vi "Query Capabilities (Voltage).vi"(0 "VISA resource name":refnum<visa-resource-name>, 5 "Absolute Maximums (T)":bool=TRUE, 11 "error in (no error)":errorcluster) -> (4 "VISA resource name out":refnum<visa-resource-name>, 6 "Voltage Capabilities":T1, 15 "error out":errorcluster)   [LabVIEW 2012, in "NH Research Regenerative Test Series.lvlib"]
doc: "Returns various Voltage capabilities of the module."
uses:
  <instrlib>/NH Research Regenerative Test Series/NH Research Regenerative Test Series.lvlib
  <instrlib>/NH Research Regenerative Test Series/Public/Utility/Voltage Capabilities.ctl
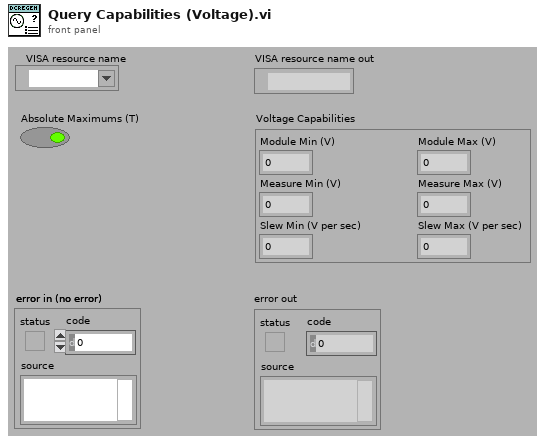
[diagram p1: front panel]
types:
  T1 = typedef "NH Research Regenerative Test Series.lvlib/Voltage Capabilities.ctl" = cluster{"Module Min (V)":dbl, "Module Max (V)":dbl, "Measure Min (V)":dbl, "Measure Max (V)":dbl, "Slew Min (V per sec)":dbl, "Slew Max (V per sec)":dbl}
  T2 = cluster{"[0]":dbl, "[1]":dbl, "[2]":dbl, "[3]":dbl, "[4]":dbl, "[5]":dbl}
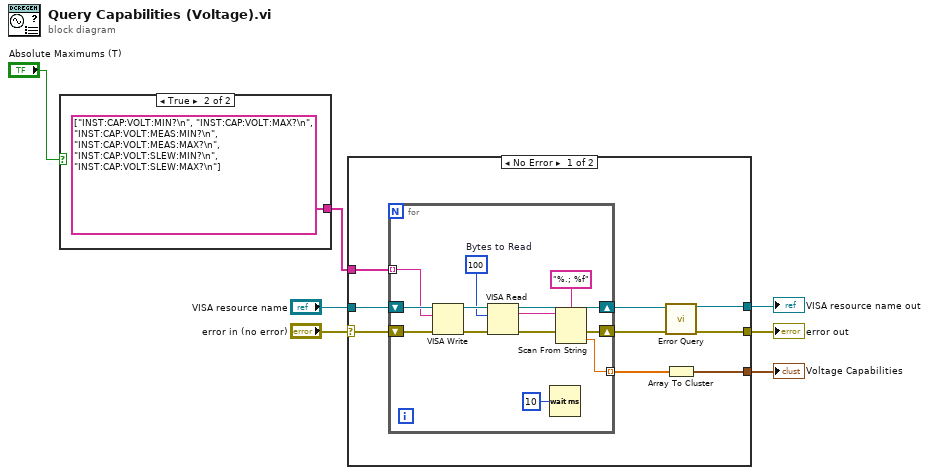
[diagram p0: block diagram]
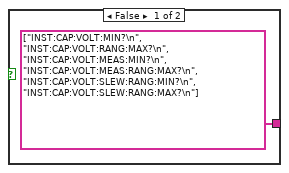
[diagram p2: hidden frame]
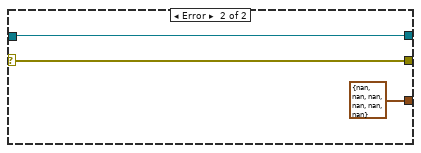
[diagram p3: hidden frame]
diagram:
  n1 = case shown="True" "Absolute Maximums (T)" {
    tunnel: [string[] ["INST:CAP:VOLT:MIN?\n", "INST:CAP:VOLT:RANG:MAX?\n", "INST:CAP:VOLT:MEAS:MIN?\n", "INST:CAP:VOLT:MEAS:RANG:MAX?\n", "INST:CAP:VOLT:SLEW:RANG:MIN?\n", "INST:CAP:VOLT:SLEW:RANG:MAX?\n"] string[] ["INST:CAP:VOLT:MIN?\n", "INST:CAP:VOLT:MAX?\n", "INST:CAP:VOLT:MEAS:MIN?\n", "INST:CAP:VOLT:MEAS:MAX?\n", "INST:CAP:VOLT:SLEW:MIN?\n", "INST:CAP:VOLT:SLEW:MAX?\n"]] -> w3
    frame False {
    }
    frame True {
    }
  }
  n2 = case shown="No Error" "error in (no error)" {
    selector: "error in (no error)" -> [w17 w34]
    tunnel: [w12 w34] -> w6
    tunnel: [w18 w33] -> w4
    tunnel: "VISA resource name" -> [w16 w33]
    tunnel: w3 -> [w15 _]
    tunnel: [w11 T1 {"Module Min (V)"=nan, "Module Max (V)"=nan, "Measure Min (V)"=nan, "Measure Max (V)"=nan, "Slew Min (V per sec)"=nan, "Slew Max (V per sec)"=nan}] -> w2
    frame No Error {
      n3 = for {
        tunnel: w15 -> [w26] mode=indexing
        tunnel: [w22] -> w14 mode=indexing
        shift-right: [w21] -> w13
        shift-left: w17 -> [w28]
        shift-right: [w20] -> w10
        shift-left: w16 -> [w27]
        w29 = u32 100  # Bytes to Read
        n4 = VISA Write(VISA resource name=w27, write buffer=w26, error in (no error)=w28) -> (VISA resource name out=w30:refnum<visa-resource-name>, error out=w31:errorcluster)  [unwired: 1 out]
        n5 = VISA Read(VISA resource name=w30, byte count=w29, error in (no error)=w31) -> (VISA resource name out=w20:refnum<visa-resource-name>, read buffer=w23:string, error out=w24:errorcluster)  [unwired: 1 out]
        n6 = Wait (ms)(milliseconds to wait=u32 10) -> ()  [unwired: 1 out]
        n7 = Scan From String(format string="%.; %f", input string=w23, error in=w24) -> (error out=w21:errorcluster, output 1=w22:dbl)  [unwired: 2 in, 2 out]
      }
      n8 = call <instrlib>:"Error Query.vi"("VISA resource name"=w10, "error in (no error)"=w13) -> ("VISA resource name out"=w18:refnum<visa-resource-name>, "error out"=w12:errorcluster)  [unwired: 10 in, 2 out]
      n9 = Array To Cluster(array=w14) -> (cluster=w11:T2)
    }
    frame Error {
    }
  }
  "error out" <- w6
  "VISA resource name out" <- w4
  "Voltage Capabilities" <- w2
